vi "Edit LDA Setup.vi"(11 "LDA info in Setup File?":bool) -> ()   [LabVIEW 2022 SP3]
uses:
  Globals/Constants_global.vi
  Globals/LDA_global.vi
panel:
  in  "String":string="Trying to Connect to Lasers.    Please Wait...."
  in  "OK":bool
  in  "LDA Setup":T1(array[cluster]) {"Req Sampling Rate Hz" min=1.0; "Shifted mW" format="%.1g"; "Unshifted mW" format="%.1g"; "Centre Velocity (m/s)" format="%.2g"; "Velocity Range (m/s)" format="%.2g"; "Centre Velocity" min=0; "Velocity Range" min=0; "Focal Length (mm)" format="%.1f"; "Beam Separation (mm)" format="%.1f"; "Lense" items=["27mm FL=300 SN=1 Actual FL=300", "27mm FL=300 SN=2 Actual FL=300", "27mm FL=160 SN=1 Actual FL=160", "27mm FL=160 SN=2 Actual FL=160", "27mm FL=160 SN=3 Actual FL=160", "27mm FL=160 SN=4 Actual FL=160", "60mm FL=500 SN=1 Actual FL=500"]; "BSA" items=["F60 SN=529 Ch=0 WL=514nm", "F60 SN=529 Ch=1 WL=488nm", "F60 SN=635 Ch=0 WL=514nm", "F60 SN=635 Ch=1 WL=488nm", "F600 SN=239 Ch=0 WL=660nm", "F600 SN=238 Ch=0 WL=532nm", "F600 SN=238 Ch=1 WL=561nm", "F600 SN=238 Ch=2 WL=553nm", "F600 SN=241 Ch=0 WL=532nm", "F600 SN=241 Ch=1 WL=561nm"]; "Laser" items=["Laser Dx_532:LAS-04839", "Laser Dx_561:LAS-05829", "FlowExplorer (660nm)", "Coherent Genesis MX (488nm)", "Coherent Genesis MX (514nm)", "Coherent Innova 70C (488nm)", "Coherent Innova 70C (514nm)"]; "Probe" items=["27mm_2D SN=141 Fibre=Green BS=14.35", "27mm_2D SN=141 Fibre=Blue BS=14.37", "27mm_2D SN=142 Fibre=Green BS=15.121", "27mm_2D SN=142 Fibre=Blue BS=15.13", "27mm_2D SN=157 Fibre=Green BS=15.47", "27mm_2D SN=157 Fibre=Blue BS=15.42", "27mm_2D SN=101 Fibre=Upper BS=15", "27mm_2D SN=101 Fibre=Lower BS=15", "27mm_1D SN=102 Fibre=Upper BS=15", "60mm SN=103 Fibre=Green BS=113.5", "60mm SN=103 Fibre=Blue BS=116", "FlowExploror SN=309 Fibre=Red BS=60"]; "Min Record length" items=["16", "32", "64", "128", "256", "512", "1024"]; "Optics Conversion Factor" format="%.3g"; "High voltage" min=0 max=2040 step=8; "Signal gain (dB)" min=0 max=30 step=1; "Max Record length" items=["16", "32", "64", "128", "256", "512", "1024"]; "Min Velocity" format="%.2g"; "Max Velocity" format="%.2g"; "Wavelength (nm)" format="%.1f"}
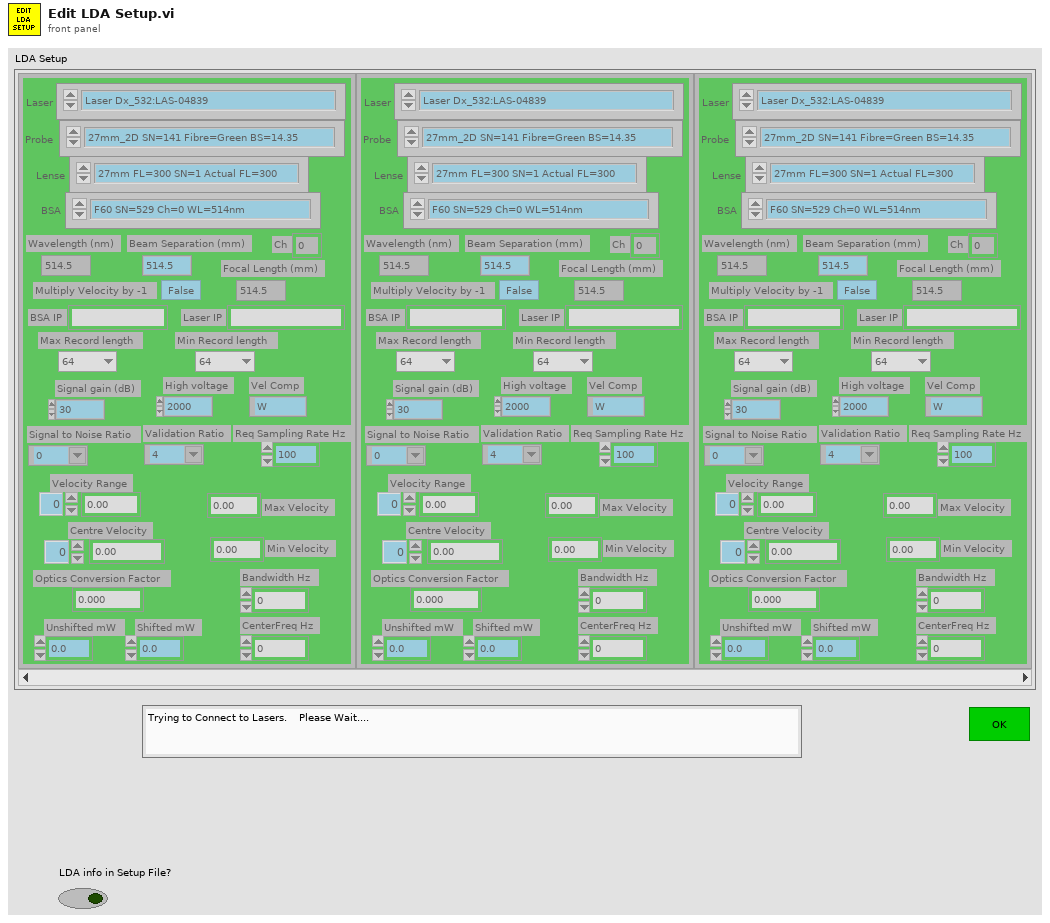
[diagram p1: front panel]
types:
  T1 = cluster{"Wavelength (nm)":dbl, "Vel Comp":string, "Max Velocity":dbl, "Min Velocity":dbl, "Max Record length":u16, "Signal gain (dB)":i16, "High voltage":i16, "Optics Conversion Factor":dbl, "Min Record length":u16, "Multiply Velocity by -1":bool, "Signal to Noise Ratio":string, "Validation Ratio":string, "Probe":u16, "Laser":u16, "BSA":u16, "Lense":u16, "Beam Separation (mm)":dbl, "Focal Length (mm)":dbl, "COLOUR":u32, "BSA IP":string, "Velocity Range":i16, "Centre Velocity":i16, "Velocity Range (m/s)":dbl, "Centre Velocity (m/s)":dbl, "Unshifted mW":dbl, "Shifted mW":dbl, "Bandwidth Hz":dbl, "Req Sampling Rate Hz":dbl, "Ch":i32, "CenterFreq Hz":dbl, "Laser IP":string}[]
  T2 = typedef "LDA_Channel.ctl" = cluster{"Wavelength (nm)":dbl, "Vel Comp":string, "Max Velocity":dbl, "Min Velocity":dbl, "Max Record length":u16, "Signal gain (dB)":i16, "High voltage":i16, "Optics Conversion Factor":dbl, "Min Record length":u16, "Multiply Velocity by -1":bool, "Signal to Noise Ratio":string, "Validation Ratio":string, "Probe":string, "Laser":string, "BSA":string, "Lense":string, "Beam Separation (mm)":dbl, "Focal Length (mm)":dbl, "COLOUR":u32, "BSA IP":string, "Velocity Range (m/s)":dbl, "Centre Velocity (m/s)":dbl, "Unshifted mW":dbl, "Shifted mW":dbl, "Bandwidth Hz":dbl, "Req Sampling Rate Hz":dbl, "Ch":i32, "CenterFreq Hz":dbl, "Laser IP":string, "Sync Delay (s)":dbl}
  T3 = cluster{"Wavelength (nm)":dbl, "Vel Comp":string, "Max Velocity":dbl, "Min Velocity":dbl, "Max Record length":u16, "Signal gain (dB)":i16, "High voltage":i16, "Optics Conversion Factor":dbl, "Min Record length":u16, "Multiply Velocity by -1":bool, "Signal to Noise Ratio":string, "Validation Ratio":string, "Probe":u16, "Laser":u16, "BSA":u16, "Lense":u16, "Beam Separation (mm)":dbl, "Focal Length (mm)":dbl, "COLOUR":u32, "BSA IP":string, "Velocity Range":i16, "Centre Velocity":i16, "Velocity Range (m/s)":dbl, "Centre Velocity (m/s)":dbl, "Unshifted mW":dbl, "Shifted mW":dbl, "Bandwidth Hz":dbl, "Req Sampling Rate Hz":dbl, "Ch":i32, "CenterFreq Hz":dbl, "Laser IP":string}
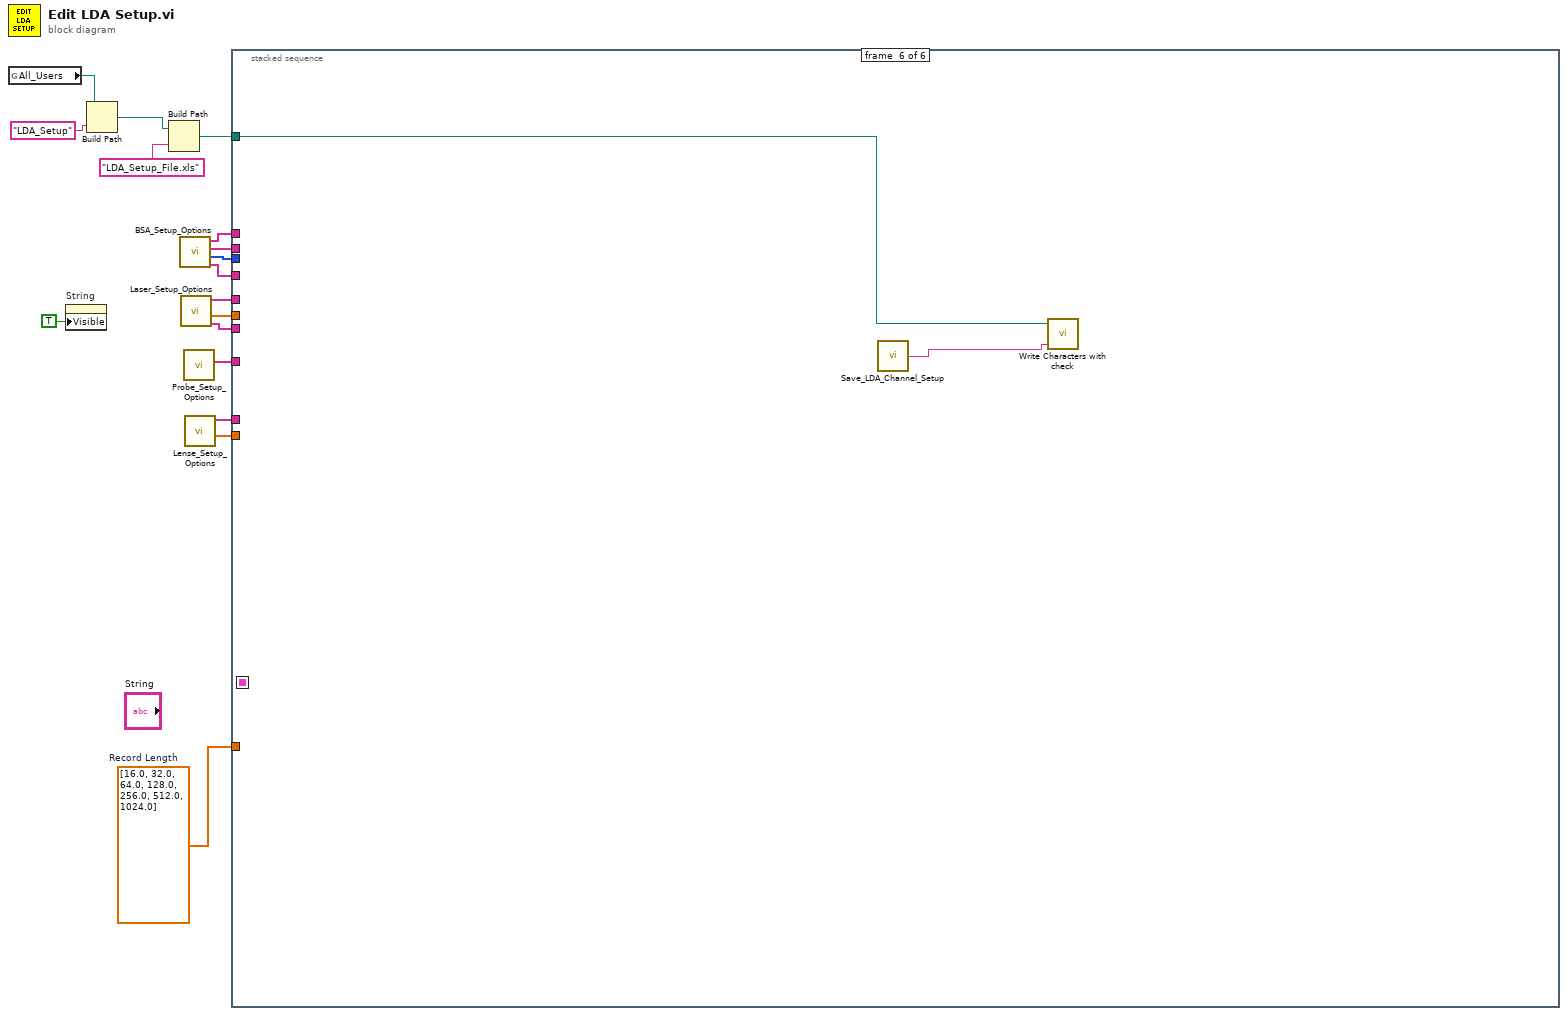
[diagram p0: block diagram]
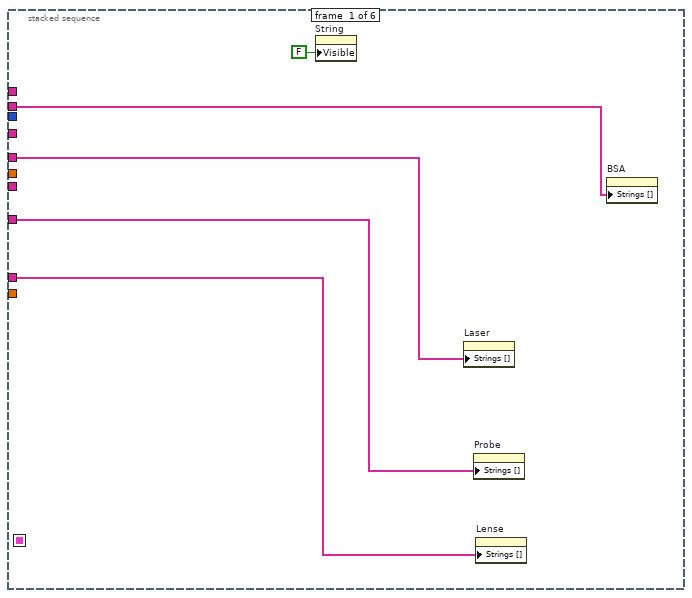
[diagram p2: hidden frame]
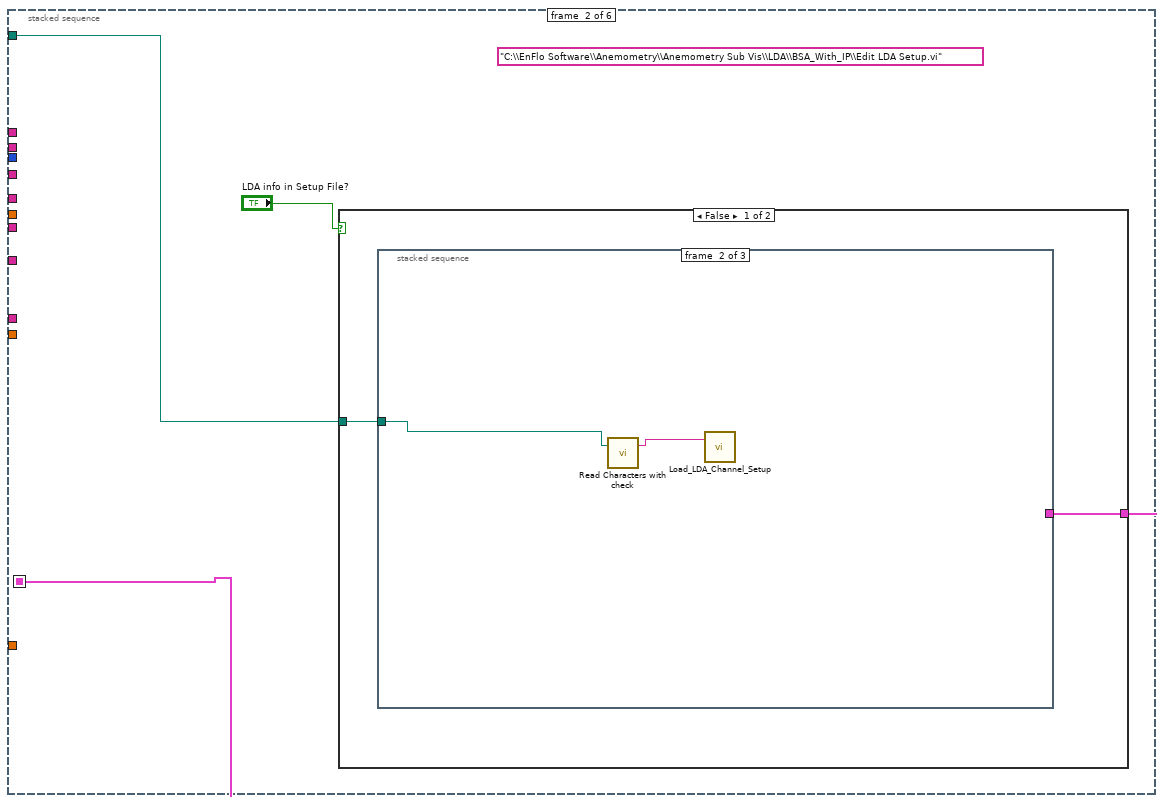
[diagram p3: hidden frame]
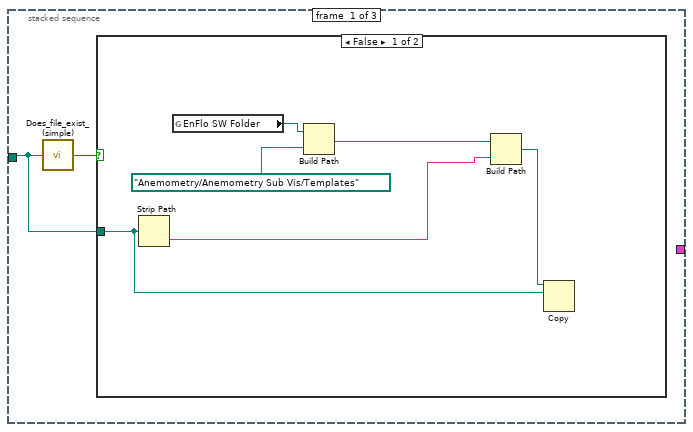
[diagram p4: hidden frame]
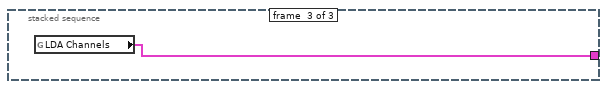
[diagram p6: hidden frame]
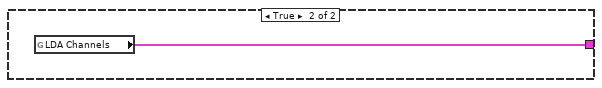
[diagram p7: hidden frame]
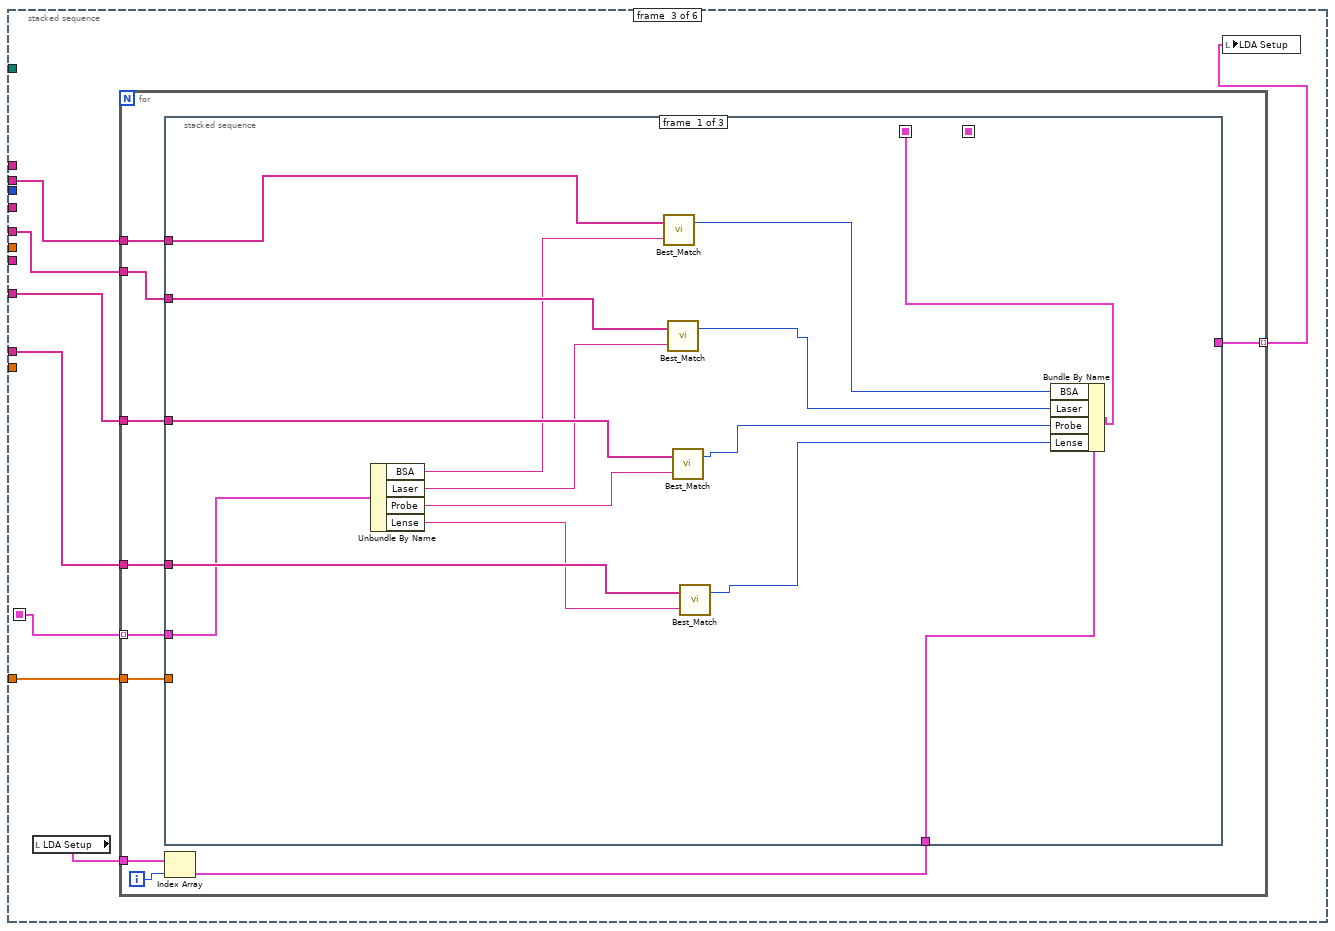
[diagram p8: hidden frame]
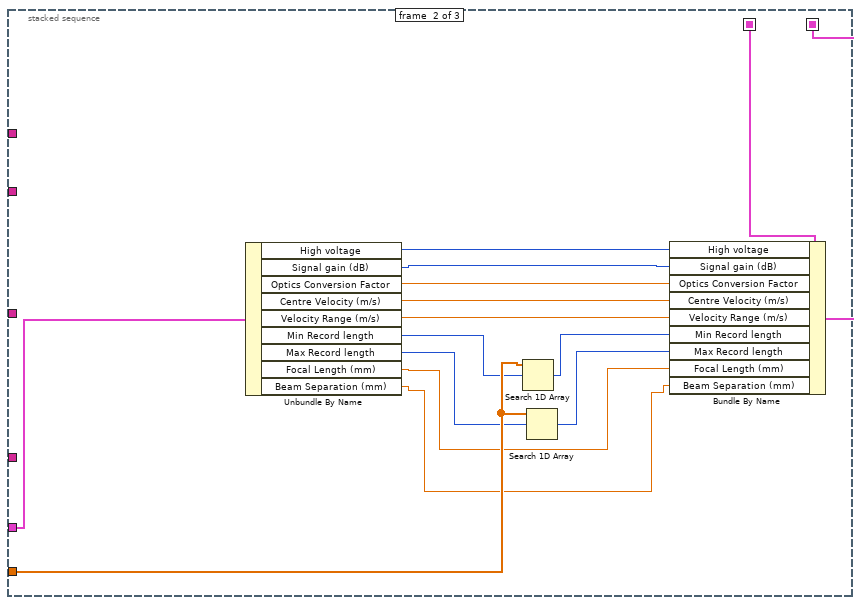
[diagram p9: hidden frame]
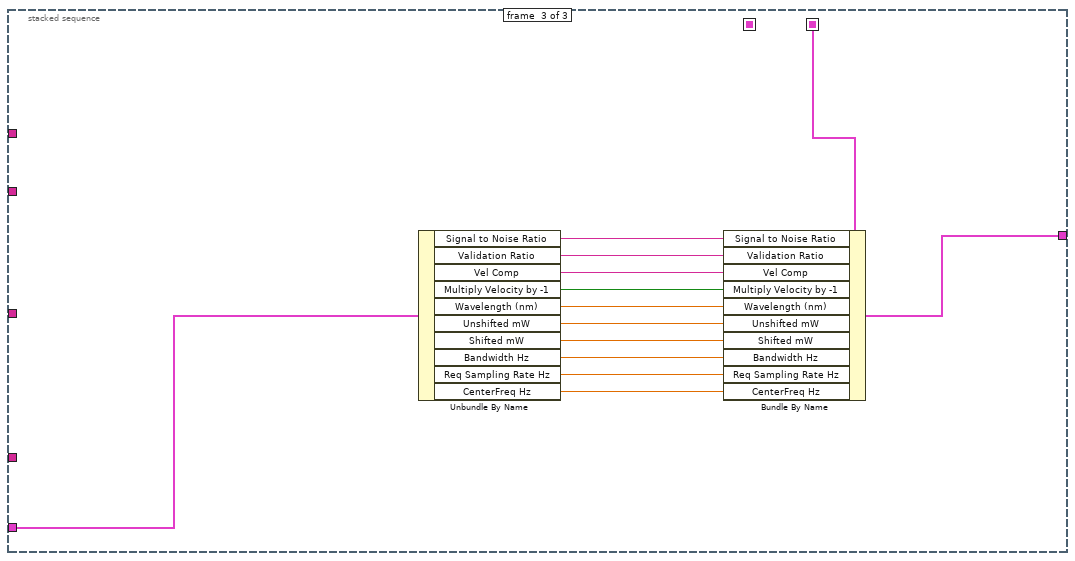
[diagram p10: hidden frame]
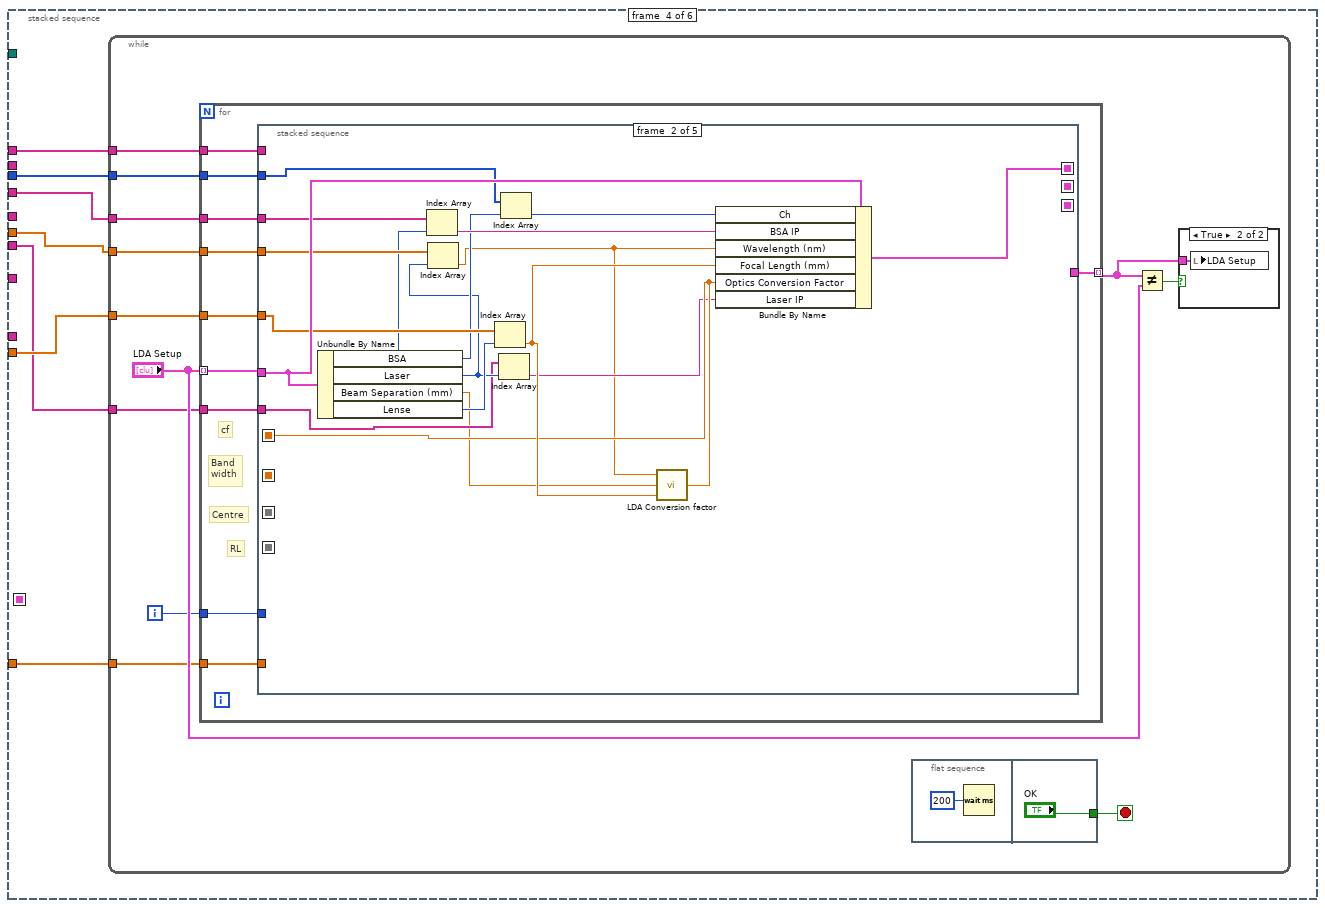
[diagram p11: hidden frame]
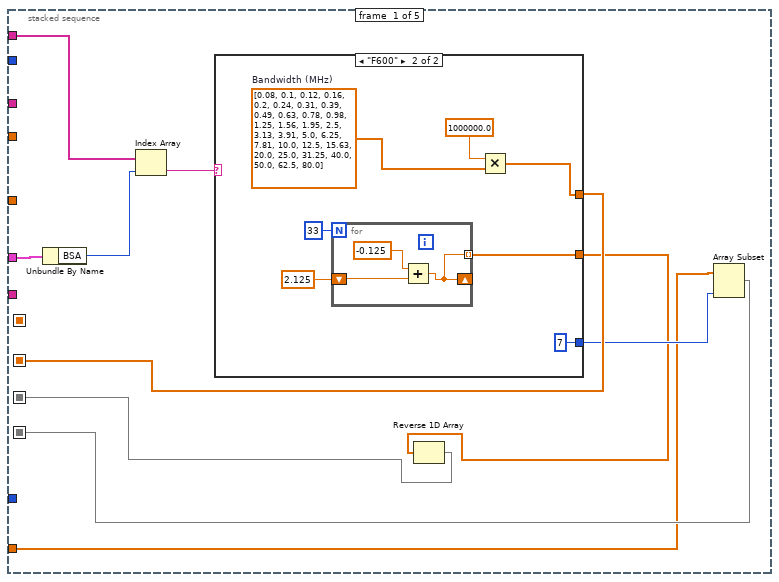
[diagram p13: hidden frame]
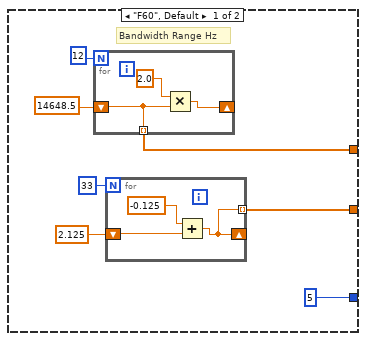
[diagram p14: hidden frame]
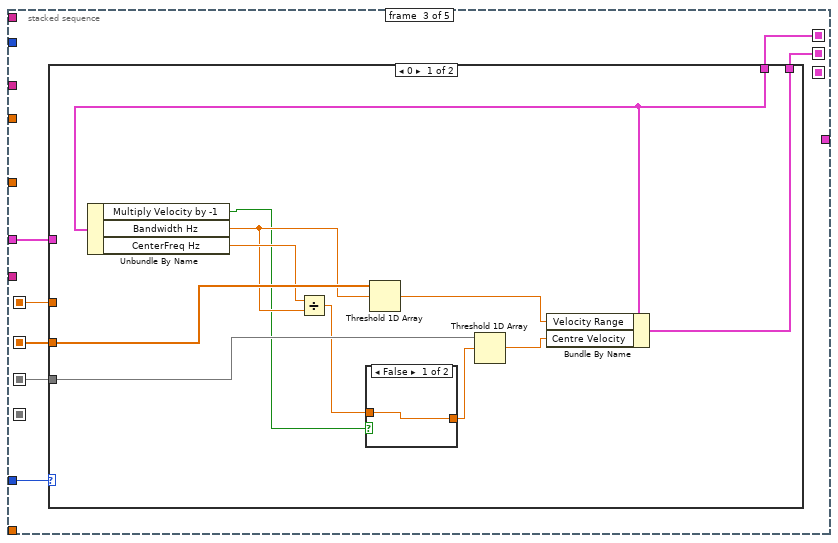
[diagram p15: hidden frame]
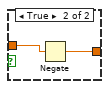
[diagram p16: hidden frame]
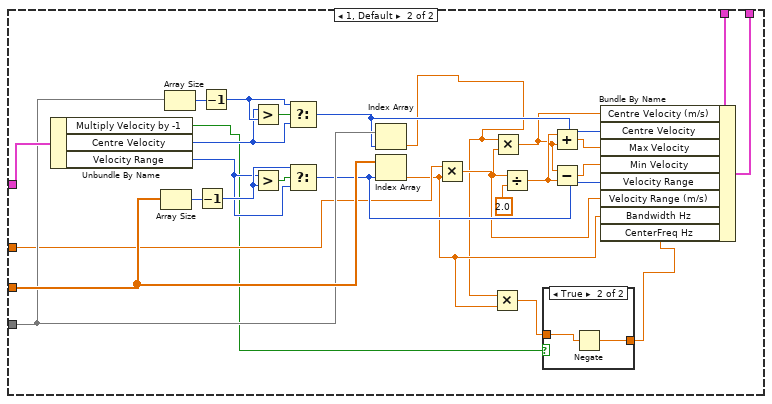
[diagram p17: hidden frame]
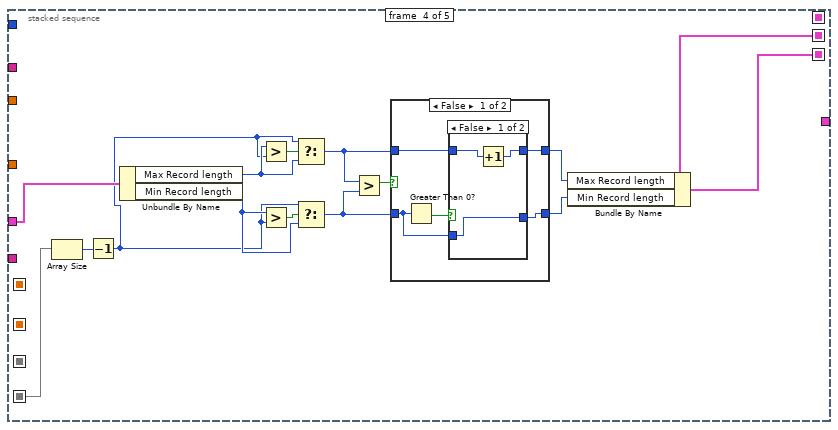
[diagram p19: hidden frame]
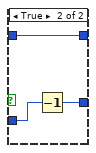
[diagram p20: hidden frame]
diagram:
  w17 = dbl[] [16.0, 32.0, 64.0, 128.0, 256.0, 512.0, 1024.0]  # Record Length
  n1 = global read "Constants_global.vi" "All_Users"() -> (w6:path)
  n2 = property on="String" class="Str"("Visible"=TRUE) -> ()  [unwired: 2 in, 2 out]
  n3 = Build Path(base path=w6, name or relative path="LDA_Setup") -> (appended path=w7:path)
  n4 = Build Path(base path=w7, name or relative path="LDA_Setup_File.xls") -> (appended path=w3:path)
  n5 = call "BSA_Setup_Options.vi"() -> ("IP Addresses"=w10:string[], "Channel Numbers"=w11:i32[], "Full BSA Strings"=w16:string[], "BSA Types"=w12:string[])  [unwired: 4 in, 1 out]
  n6 = call "Laser_Setup_Options.vi"() -> ("Lasers IP Numbers"=w2:string[], "Wavelengths"=w9:dbl[], "Lasers"=w15:string[])  [unwired: 5 in, 1 out]
  n7 = call "Probe_Setup_Options.vi"() -> ("Probes"=w14:string[])  [unwired: 8 in]
  n8 = call "Lense_Setup_Options.vi"() -> ("Focal Lengths"=w8:dbl[], "Lenses"=w13:string[])  [unwired: 7 in]
  n9 = stacked-sequence {
    seq-local: [_ w25 _ _ _ _] -> [_ _ w40 _ w267 _]
    tunnel: w17 -> [_ _ w46 w107 w271 _]
    tunnel: w16 -> [w22 _ w41 _ _ _]
    tunnel: w15 -> [w21 _ w42 _ _ _]
    tunnel: w14 -> [w20 _ w43 _ _ _]
    tunnel: w13 -> [w19 _ w44 _ _ _]
    tunnel: w12 -> [_ _ _ w106 _ _]
    tunnel: w11 -> [_ _ _ w105 _ _]
    tunnel: w10 -> [_ _ _ w104 _ _]
    tunnel: w9 -> [_ _ _ w103 _ _]
    tunnel: w8 -> [_ _ _ w102 _ _]
    tunnel: w3 -> [_ w24 _ _ _ w347]
    tunnel: w2 -> [_ _ _ w101 _ _]
    frame #0 {
      n10 = property on="String" class="Str"("Visible"=FALSE) -> ()  [unwired: 2 in, 2 out]
      n11 = property on="Laser" class="Ring (strict)"("Strings []"=w21) -> ()  [unwired: 2 in, 2 out]
      n12 = property on="Probe" class="Ring (strict)"("Strings []"=w20) -> ()  [unwired: 2 in, 2 out]
      n13 = property on="Lense" class="Ring (strict)"("Strings []"=w19) -> ()  [unwired: 2 in, 2 out]
      n14 = property on="BSA" class="Ring (strict)"("Strings []"=w22) -> ()  [unwired: 2 in, 2 out]
    }
    frame #1 {
      (unwired) "C:\\EnFlo Software\\Anemometry\\Anemometry Sub Vis\\LDA\\BSA_With_IP\\Edit LDA Setup.vi"
      n15 = case shown="False" "LDA info in Setup File?" {
        tunnel: [w26 w39] -> w25
        tunnel: w24 -> [w27 _]
        frame False {
          n16 = stacked-sequence {
            tunnel: w27 -> [w28 w37 _]
            tunnel: [_ _ w38] -> w26
            frame #0 {
              n17 = call "Does_file_exist_(simple).vi"("Pathname"=w28) -> ("exists?"=w29:bool)
              n18 = case shown="False" w29 {
                tunnel: w28 -> [w30 _]
                frame False {
                  n19 = Strip Path(path=w30) -> (name=w32:string)  [unwired: 1 out]
                  n20 = global read "Constants_global.vi" "EnFlo SW Folder"() -> (w35:path)
                  n21 = Build Path(base path=w35, name or relative path=path "Anemometry/Anemometry Sub Vis/Templates" ("appended path")) -> (appended path=w33:path)
                  n22 = Build Path(base path=w33, name or relative path=w32) -> (appended path=w31:path)
                  n23 = Copy(10:w30, 11:w31) -> ()  [unwired: 3 in, 3 out]
                }
                frame True {
                }
              }
            }
            frame #1 {
              n24 = call "Read Characters with check.vi"("file (use dialog)"=w37) -> ("Read String"=w36:string)  [unwired: 1 in, 1 out]
              n25 = call "Load_LDA_Channel_Setup.vi"("Setup file string"=w36) -> ()  [unwired: 2 in]
            }
            frame #2 {
              n26 = global read "LDA_global.vi" "LDA Channels"() -> (w38:T2[])
            }
          }
        }
        frame True {
          n27 = global read "LDA_global.vi" "LDA Channels"() -> (w39:T2[])
        }
      }
    }
    frame #2 {
      n28 = local read "LDA Setup"() -> (w47:T1)
      n29 = for {
        tunnel: w47 -> [w57]
        tunnel: w46 -> [w54]
        tunnel: [w53] -> w45 mode=indexing
        tunnel: w41 -> [w52]
        tunnel: w42 -> [w51]
        tunnel: w43 -> [w50]
        tunnel: w44 -> [w49]
        tunnel: w40 -> [w48] mode=indexing
        i -> [w56]
        n30 = Index Array(array=w57, index=w56) -> (element=w55:T3)
        n31 = stacked-sequence {
          seq-local: [w67 _ _] -> [_ w84 _]
          seq-local: [_ w83 _] -> [_ _ w100]
          tunnel: w55 -> [w72 _ _]
          tunnel: w54 -> [_ w86 _]
          tunnel: [_ _ w99] -> w53
          tunnel: w52 -> [w66 _ _]
          tunnel: w51 -> [w65 _ _]
          tunnel: w50 -> [w64 _ _]
          tunnel: w49 -> [w63 _ _]
          tunnel: w48 -> [w62 w82 w91]
          frame #0 {
            n32 = Unbundle By Name(w62) -> ("BSA"=w61:string, "Laser"=w60:string, "Probe"=w59:string, "Lense"=w58:string)
            n33 = call "Best_Match.vi"("Input String"=w61, "String Options"=w66) -> ("index of element"=w71:i32)  [unwired: 1 out]
            n34 = call "Best_Match.vi"("Input String"=w60, "String Options"=w65) -> ("index of element"=w70:i32)  [unwired: 1 out]
            n35 = call "Best_Match.vi"("Input String"=w59, "String Options"=w64) -> ("index of element"=w69:i32)  [unwired: 1 out]
            n36 = call "Best_Match.vi"("Input String"=w58, "String Options"=w63) -> ("index of element"=w68:i32)  [unwired: 1 out]
            n37 = Bundle By Name(cluster=w72, "BSA"=w71, "Laser"=w70, "Probe"=w69, "Lense"=w68) -> (w67:T3)
          }
          frame #1 {
            n38 = Unbundle By Name(w82) -> ("High voltage"=w81:i16, "Signal gain (dB)"=w80:i16, "Optics Conversion Factor"=w79:dbl, "Centre Velocity (m/s)"=w78:dbl, "Velocity Range (m/s)"=w77:dbl, "Min Record length"=w76:u16, "Max Record length"=w75:u16, "Focal Length (mm)"=w74:dbl, "Beam Separation (mm)"=w73:dbl)
            n39 = Search 1D Array(1D array=w86, element=w76) -> (index of element=w85:i32)  [unwired: 1 in]
            n40 = Search 1D Array(1D array=w86, element=w75) -> (index of element=w87:i32)  [unwired: 1 in]
            n41 = Bundle By Name(cluster=w84, "High voltage"=w81, "Signal gain (dB)"=w80, "Optics Conversion Factor"=w79, "Centre Velocity (m/s)"=w78, "Velocity Range (m/s)"=w77, "Min Record length"=w85, "Max Record length"=w87, "Focal Length (mm)"=w74, "Beam Separation (mm)"=w73) -> (w83:T3)
          }
          frame #2 {
            n42 = Unbundle By Name(w91) -> ("Signal to Noise Ratio"=w98:string, "Validation Ratio"=w97:string, "Vel Comp"=w96:string, "Multiply Velocity by -1"=w95:bool, "Wavelength (nm)"=w94:dbl, "Unshifted mW"=w93:dbl, "Shifted mW"=w92:dbl, "Bandwidth Hz"=w90:dbl, "Req Sampling Rate Hz"=w88:dbl, "CenterFreq Hz"=w89:dbl)
            n43 = Bundle By Name(cluster=w100, "Signal to Noise Ratio"=w98, "Validation Ratio"=w97, "Vel Comp"=w96, "Multiply Velocity by -1"=w95, "Wavelength (nm)"=w94, "Unshifted mW"=w93, "Shifted mW"=w92, "Bandwidth Hz"=w90, "Req Sampling Rate Hz"=w88, "CenterFreq Hz"=w89) -> (w99:T3)
          }
        }
      }
      n44 = local write "LDA Setup"(w45) -> ()
    }
    frame #3 {
      n45 = while {
        tunnel: w104 -> [w119]
        tunnel: w103 -> [w118]
        tunnel: w102 -> [w117]
        tunnel: w106 -> [w112]
        tunnel: w107 -> [w111]
        tunnel: w105 -> [w110]
        tunnel: w101 -> [w108]
        i -> [w109]
        stop <- w116 stop-if-true
        n46 = for {
          tunnel: "LDA Setup" -> [w132] mode=indexing
          tunnel: w119 -> [w131]
          tunnel: w118 -> [w130]
          tunnel: w117 -> [w129]
          tunnel: [w128] -> w113 mode=indexing
          tunnel: w112 -> [w127]
          tunnel: w111 -> [w126]
          tunnel: w110 -> [w125]
          tunnel: w109 -> [w124]
          tunnel: w108 -> [w123]
          # "RL"
          # "cf"
          # "Band\nwidth"
          # "Centre"
          n47 = stacked-sequence {
            seq-local: [w138 _ _ _ _] -> [_ _ w187 _ _]
            seq-local: [w134 _ _ _ _] -> [_ _ w186 _ _]
            seq-local: [_ w175 _ _ _] -> [_ _ w185 _ _]
            seq-local: [_ w174 _ _ _] -> [_ _ w188 _ _]
            seq-local: [_ _ w184 _ _] -> [_ _ _ w242 _]
            seq-local: [w137 _ _ _ _] -> [_ _ _ w240 _]
            seq-local: [_ _ _ w241 _] -> [_ _ _ _ w262]
            tunnel: w132 -> [w142 w182 w189 w248 w266]
            tunnel: w131 -> [_ w181 _ _ _]
            tunnel: w130 -> [_ w180 _ _ _]
            tunnel: w129 -> [_ w179 _ _ _]
            tunnel: [_ _ _ _ w263] -> w128
            tunnel: w127 -> [w140 _ _ _ _]
            tunnel: w126 -> [w135 _ _ _ _]
            tunnel: w125 -> [_ w171 _ _ _]
            tunnel: w124 -> [_ _ w183 _ _]
            tunnel: w123 -> [_ w169 _ _ _]
            frame #0 {
              n48 = Unbundle By Name(w142) -> ("BSA"=w141:u16)
              n49 = Index Array(array=w140, index=w141) -> (element=w139:string)
              n50 = case shown="\"F600\"" w139 {
                tunnel: [w145 w160] -> w133
                tunnel: [w144 w156] -> w138
                tunnel: [5 ("length") 7 ("length")] -> w136
                frame "F60", Default {
                  # "Bandwidth Range Hz"
                  n51 = for {
                    N: 12 -> [_]
                    shift-right: [w155] -> _
                    shift-left: 14648.5 -> [w153]
                    tunnel: [w153] -> w144 mode=indexing
                    n52 = Multiply(x=2.0, y=w153) -> (x*y=w155:dbl)
                  }
                  n53 = for {
                    N: 33 -> [_]
                    shift-right: [w150] -> _
                    shift-left: 2.125 -> [w152]
                    tunnel: [w150] -> w145 mode=indexing
                    n54 = Add(x=-0.125, y=w152) -> (x+y=w150:dbl)
                  }
                }
                frame "F600" {
                  w158 = dbl[] [0.08, 0.1, 0.12, 0.16, 0.2, 0.24, 0.31, 0.39, 0.49, 0.63, 0.78, 0.98, 1.25, 1.56, 1.95, 2.5, 3.13, 3.91, 5.0, 6.25, 7.81, 10.0, 12.5, 15.63, 20.0, 25.0, 31.25, 40.0, 50.0, 62.5, 80.0]  # Bandwidth (MHz)
                  n55 = for {
                    N: 33 -> [_]
                    shift-right: [w163] -> _
                    shift-left: 2.125 -> [w165]
                    tunnel: [w163] -> w160 mode=indexing
                    n56 = Add(x=-0.125, y=w165) -> (x+y=w163:dbl)
                  }
                  n57 = Multiply(x=1000000.0, y=w158) -> (x*y=w156:dbl[])
                }
              }
              n58 = Reverse 1D Array(array=w133) -> (reversed array=w134:dbl[])
              n59 = Array Subset(array=w135, length=w136) -> (w137:dbl[])  [unwired: 1 in]
            }
            frame #1 {
              n60 = Unbundle By Name(w182) -> ("BSA"=w173:u16, "Laser"=w170:u16, "Beam Separation (mm)"=w167:dbl, "Lense"=w178:u16)
              n61 = Index Array(array=w181, index=w173) -> (element=w176:string)
              n62 = Index Array(array=w180, index=w170) -> (element=w166:dbl)
              n63 = Index Array(array=w179, index=w178) -> (element=w177:dbl)
              n64 = Index Array(array=w169, index=w170) -> (element=w168:string)
              n65 = Index Array(array=w171, index=w173) -> (element=w172:i32)
              n66 = call "LDA Conversion factor.vi"("Focal Length"=w177, "Beam Separation (mm)"=w167, "Wavelength (nm)"=w166) -> ("cf"=w175:dbl)
              n67 = Bundle By Name(cluster=w182, "Ch"=w172, "BSA IP"=w176, "Wavelength (nm)"=w166, "Focal Length (mm)"=w177, "Optics Conversion Factor"=w175, "Laser IP"=w168) -> (w174:T3)
            }
            frame #2 {
              n68 = case shown="0" w183 {
                tunnel: w189 -> [_ w230]
                tunnel: w188 -> [w197 w228]
                tunnel: w187 -> [w200 w224]
                tunnel: w186 -> [w199 w216]
                tunnel: w185 -> [_ w212]
                tunnel: [w196 w209] -> w184
                frame 0 {
                  n69 = Unbundle By Name(w197) -> ("Multiply Velocity by -1"=w191:bool, "Bandwidth Hz"=w194:dbl, "CenterFreq Hz"=w195:dbl)
                  n70 = Divide(x=w195, y=w194) -> (x/y=w192:dbl)
                  n71 = case shown="False" w191 {
                    tunnel: w192 -> [w201 w203]
                    tunnel: [w201 w202] -> w190
                    frame False {
                    }
                    frame True {
                      n72 = Negate(x=w203) -> (-x=w202:dbl)
                    }
                  }
                  n73 = Threshold 1D Array(2:w194, 3:w200) -> (0:w198:dbl)  [unwired: 1 in]
                  n74 = Threshold 1D Array(2:w190, 3:w199) -> (0:w193:dbl)  [unwired: 1 in]
                  n75 = Bundle By Name(cluster=w197, "Velocity Range"=w198, "Centre Velocity"=w193) -> (w196:T3)
                }
                frame 1, Default {
                  n76 = Unbundle By Name(w230) -> ("Multiply Velocity by -1"=w206:bool, "Centre Velocity"=w213:i16, "Velocity Range"=w220:i16)
                  n77 = Array Size(array=w224) -> (size(s)=w223:i32)
                  n78 = Array Size(array=w216) -> (size(s)=w217:i32)
                  n79 = Decrement(x=w223) -> (x-1=w221:i32)
                  n80 = Decrement(x=w217) -> (x-1=w219:i32)
                  n81 = Greater?(x=w213, y=w219) -> (0:w218:bool)
                  n82 = Greater?(x=w220, y=w221) -> (0:w222:bool)
                  n83 = Select(t=w219, s=w218, f=w213) -> (s? t:f=w215:i32)
                  n84 = Select(t=w221, s=w222, f=w220) -> (s? t:f=w214:i32)
                  n85 = Index Array(array=w216, index=w215) -> (element=w207:dbl)
                  n86 = Index Array(array=w224, index=w214) -> (element=w208:dbl)
                  n87 = Multiply(x=w212, y=w208) -> (x*y=w211:dbl)
                  n88 = Multiply(x=w207, y=w208) -> (x*y=w205:dbl)
                  n89 = Multiply(x=w207, y=w211) -> (x*y=w210:dbl)
                  n90 = Divide(x=w211, y=2.0) -> (x/y=w226:dbl)
                  n91 = case shown="True" w206 {
                    tunnel: w205 -> [w231 w233]
                    tunnel: [w231 w232] -> w204
                    frame False {
                    }
                    frame True {
                      n92 = Negate(x=w233) -> (-x=w232:dbl)
                    }
                  }
                  n93 = Add(x=w226, y=w210) -> (x+y=w227:dbl)
                  n94 = Subtract(x=w210, y=w226) -> (x-y=w225:dbl)
                  n95 = Bundle By Name(cluster=w228, "Centre Velocity (m/s)"=w210, "Centre Velocity"=w215, "Max Velocity"=w227, "Min Velocity"=w225, "Velocity Range"=w214, "Velocity Range (m/s)"=w211, "Bandwidth Hz"=w208, "CenterFreq Hz"=w204) -> (w209:T3)
                }
              }
            }
            frame #3 {
              n96 = Array Size(array=w240) -> (size(s)=w247:i32)
              n97 = Decrement(x=w247) -> (x-1=w234:i32)
              n98 = Unbundle By Name(w248) -> ("Max Record length"=w243:u16, "Min Record length"=w245:u16)
              n99 = Greater?(x=w243, y=w234) -> (0:w244:bool)
              n100 = Greater?(x=w245, y=w234) -> (0:w246:bool)
              n101 = Select(t=w234, s=w244, f=w243) -> (s? t:f=w237:i32)
              n102 = Select(t=w234, s=w246, f=w245) -> (s? t:f=w235:i32)
              n103 = Greater?(x=w237, y=w235) -> (0:w239:bool)
              n104 = case shown="False" w239 {
                tunnel: [w249 w261] -> w238
                tunnel: w237 -> [w250 w261]
                tunnel: [w251 w260] -> w236
                tunnel: w235 -> [w252 w260]
                frame False {
                  n105 = Greater Than 0?(x=w252) -> (x > 0?=w253:bool)
                  n106 = case shown="False" w253 {
                    tunnel: w252 -> [w256 w259]
                    tunnel: [w256 w258] -> w251
                    tunnel: w250 -> [w254 w257]
                    tunnel: [w255 w257] -> w249
                    frame False {
                      n107 = Increment(x=w254) -> (x+1=w255:i32)
                    }
                    frame True {
                      n108 = Decrement(x=w259) -> (x-1=w258:i32)
                    }
                  }
                }
                frame True {
                }
              }
              n109 = Bundle By Name(cluster=w242, "Max Record length"=w238, "Min Record length"=w236) -> (w241:T3)
            }
            frame #4 {
              n110 = Unbundle By Name(w266) -> ("Wavelength (nm)"=w265:dbl)
              n111 = call "wavelength to color.vi"("Wavelength (380 - 780)"=w265) -> ("Color"=w264:u32)  [unwired: 1 out]
              n112 = Bundle By Name(cluster=w262, "COLOUR"=w264) -> (w263:T3)
            }
          }
        }
        n113 = flat-sequence {
          tunnel: ["OK"] -> w116
          frame #0 {
            n114 = Wait (ms)(milliseconds to wait=u32 200) -> ()  [unwired: 1 out]
          }
          frame #1 {
          }
        }
        n115 = Not Equal?(x=w113, y="LDA Setup") -> (x != y?=w114:bool)
        n116 = case shown="True" w114 {
          tunnel: w113 -> [_ w120]
          frame False {
          }
          frame True {
            n117 = local write "LDA Setup"(w120) -> ()
          }
        }
      }
    }
    frame #4 {
      n118 = local read "LDA Setup"() -> (w272:T1)
      n119 = Index Array(array=w267, index=0) -> (element=w269:T2)
      n120 = for {
        tunnel: w272 -> [w278] mode=indexing
        tunnel: w271 -> [w275]
        tunnel: w269 -> [w274]
        tunnel: [w273] -> w268 mode=indexing
        i -> [w277]
        n121 = Increment(x=w277) -> (x+1=w276:i32)
        n122 = stacked-sequence {
          seq-local: [w285 _ _ _ _] -> [_ _ _ _ _]
          seq-local: [w279 _ _ _ _] -> [_ w315 _ _ _]
          seq-local: [_ w307 _ _ _] -> [_ _ w327 _ _]
          seq-local: [_ _ w321 _ _] -> [_ _ _ w333 _]
          seq-local: [_ _ _ w332 _] -> [_ _ _ _ w339]
          tunnel: w278 -> [w306 w319 w328 w336 w345]
          tunnel: w276 -> [w302 _ _ _ _]
          tunnel: w275 -> [_ w316 _ _ _]
          tunnel: w274 -> [w284 _ _ _ _]
          tunnel: [_ _ _ _ w340] -> w273
          frame #0 {
            n123 = Number To Decimal String(number=w302) -> (decimal integer string=w305:string)  [unwired: 1 out]
            n124 = Unbundle By Name(w306) -> ("Probe"=w296:u16, "Laser"=w294:u16, "BSA"=w286:u16, "Lense"=w287:u16)
            n125 = Concatenate Strings("BSA ", w305, " ") -> (w285:string)
            n126 = property on="Lense" class="Ring (strict)"() -> ("Strings []"=w288:string[])  [unwired: 2 in, 2 out]
            n127 = property on="Probe" class="Ring (strict)"() -> ("Strings []"=w297:string[])  [unwired: 2 in, 2 out]
            n128 = property on="Laser" class="Ring (strict)"() -> ("Strings []"=w295:string[])  [unwired: 2 in, 2 out]
            n129 = property on="BSA" class="Ring (strict)"() -> ("Strings []"=w289:string[])  [unwired: 2 in, 2 out]
            n130 = Index Array(array=w295, index=w294) -> (element=w281:string)
            n131 = Index Array(array=w289, index=w286) -> (element=w282:string)
            n132 = Index Array(array=w288, index=w287) -> (element=w283:string)
            n133 = Index Array(array=w297, index=w296) -> (element=w280:string)
            n134 = Concatenate Strings(w285, "Probe_Info" ("Pre Setup String")) -> (w299:string)
            n135 = Concatenate Strings(w285, "Laser_Info" ("string")) -> (w300:string)
            n136 = Concatenate Strings(w285, "BSA_Info" ("string")) -> (w293:string)
            n137 = Concatenate Strings(w285, "Lense_Info" ("string")) -> (w290:string)
            n138 = call "Characters_to_string.vi"("Characters to write"=w281, "Label for characters"=w300) -> ()  [unwired: 1 in, 1 out]
            n139 = call "Characters_to_string.vi"("Characters to write"=w280, "Label for characters"=w299) -> ()  [unwired: 1 in, 1 out]
            n140 = call "Characters_to_string.vi"("Characters to write"=w282, "Label for characters"=w293) -> ()  [unwired: 1 in, 1 out]
            n141 = call "Characters_to_string.vi"("Characters to write"=w283, "Label for characters"=w290) -> ()  [unwired: 1 in, 1 out]
            n142 = Bundle By Name(cluster=w284, "Probe"=w280, "Laser"=w281, "BSA"=w282, "Lense"=w283) -> (w279:T2)
          }
          frame #1 {
            n143 = Unbundle By Name(w319) -> ("Optics Conversion Factor"=w314:dbl, "Centre Velocity (m/s)"=w313:dbl, "Velocity Range (m/s)"=w312:dbl, "Min Record length"=w318:u16, "Max Record length"=w317:u16, "Focal Length (mm)"=w309:dbl, "Beam Separation (mm)"=w308:dbl)
            n144 = Index Array(array=w316, index=w318) -> (element=w311:dbl)
            n145 = Index Array(array=w316, index=w317) -> (element=w310:dbl)
            n146 = Bundle By Name(cluster=w315, "Optics Conversion Factor"=w314, "Centre Velocity (m/s)"=w313, "Velocity Range (m/s)"=w312, "Min Record length"=w311, "Max Record length"=w310, "Focal Length (mm)"=w309, "Beam Separation (mm)"=w308) -> (w307:T2)
          }
          frame #2 {
            n147 = Unbundle By Name(w328) -> ("BSA IP"=w320:string, "Vel Comp"=w326:string, "Multiply Velocity by -1"=w325:bool, "Wavelength (nm)"=w324:dbl, "High voltage"=w323:i16, "Signal gain (dB)"=w322:i16)
            n148 = Bundle By Name(cluster=w327, "BSA IP"=w320, "Vel Comp"=w326, "Multiply Velocity by -1"=w325, "Wavelength (nm)"=w324, "High voltage"=w323, "Signal gain (dB)"=w322) -> (w321:T2)
          }
          frame #3 {
            n149 = Unbundle By Name(w336) -> ("Ch"=w329:i32, "Bandwidth Hz"=w335:dbl, "CenterFreq Hz"=w334:dbl, "Max Velocity"=w331:dbl, "Min Velocity"=w330:dbl)
            n150 = Bundle By Name(cluster=w333, "Ch"=w329, "Bandwidth Hz"=w335, "CenterFreq Hz"=w334, "Max Velocity"=w331, "Min Velocity"=w330) -> (w332:T2)
          }
          frame #4 {
            n151 = Unbundle By Name(w345) -> ("Req Sampling Rate Hz"=w338:dbl, "Signal to Noise Ratio"=w344:string, "Validation Ratio"=w343:string, "Unshifted mW"=w342:dbl, "Shifted mW"=w341:dbl, "Laser IP"=w337:string)
            n152 = Bundle By Name(cluster=w339, "Req Sampling Rate Hz"=w338, "Signal to Noise Ratio"=w344, "Validation Ratio"=w343, "Unshifted mW"=w342, "Shifted mW"=w341, "Laser IP"=w337) -> (w340:T2)
          }
        }
      }
      n153 = global write "LDA_global.vi" "LDA Channels"(w268) -> ()
    }
    frame #5 {
      n154 = call "Save_LDA_Channel_Setup.vi"() -> ("Setup file string"=w346:string)  [unwired: 1 in]
      n155 = call "Write Characters with check.vi"("String to Write"=w346, "file (use dialog)"=w347) -> ()  [unwired: 2 in, 1 out]
    }
  }
